vi "Clear Arbitrary Waveform.vi"(7 "Clear All Waveforms (False)":bool, 8 "error in (no error)":errorcluster, 10 "Arbitrary Waveform Name":string, 11 "VISA resource name":refnum<visa-resource-name>) -> (0 "error out":errorcluster, 3 "VISA resource name out":refnum<visa-resource-name>)   [LabVIEW 2020, in "Template - Function Generator.lvlib"]
doc: "Removes a previously created arbitrary waveform from the function generator's memory."
uses:
  <instrlib>/_Template - Function Generator/Template - Function Generator.lvlib
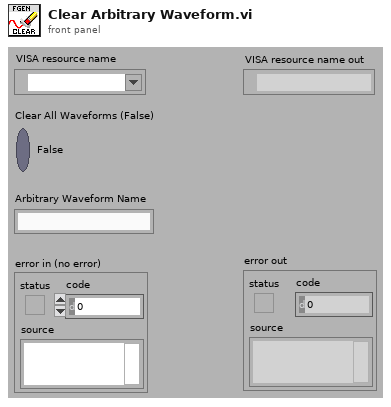
[diagram p1: front panel]
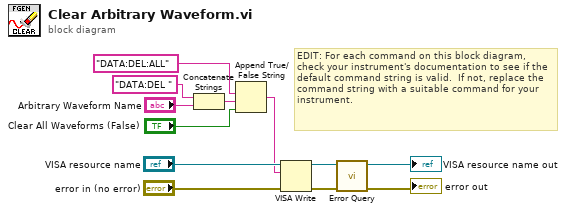
[diagram p0: block diagram]
diagram:
  # "EDIT: For each command on this block diagram, check your instrument's documentation to see if the default command string is valid.  If not, replace the command string with a suitable command for your instrument."
  n1 = Concatenate Strings("DATA:DEL " ("string"), "Arbitrary Waveform Name") -> (w8:string)
  n2 = Append True/False String(1:"Clear All Waveforms (False)", 2:w8, 3:"DATA:DEL:ALL" ("true string")) -> (0:w5:string)  [unwired: 1 in]
  n3 = VISA Write(VISA resource name="VISA resource name", write buffer=w5, error in (no error)="error in (no error)") -> (VISA resource name out=w4:refnum<visa-resource-name>, error out=w2:errorcluster)  [unwired: 1 out]
  n4 = call <instrlib>:"Error Query.vi"("error in (no error)"=w2, "VISA resource name"=w4) -> ("error out"=→"error out":errorcluster, "VISA resource name out"=→"VISA resource name out":refnum<visa-resource-name>)  [unwired: 6 in, 2 out]
